vi "camera acquisition.vi"(0 "Interface Name":string="cam0", 9 "Stop (F)":bool, 11 "error in":errorcluster) -> (4 "Image Out":T1(plugin-control), 6 "Frame Rate":dbl, 8 "Image Number":u32, 10 "Stopped":bool, 15 "error out":errorcluster)   [LabVIEW 2020]
doc: "Creates, and edits acquisitions using the NI Vision Acquisition Express VI.\n\nThe NI Vision Acquisition Wizard is launched by placing the Express VI on the block diagram. Select an acquisition source and configure an acquisition using NI-IMAQ, NI-IMAQdx, or simulate an acquisition by reading an AVI or image files from a folder. After an acquisition is configured, select controls and indicators to be able to programmatically set in LabVIEW. Double-click the Vision Acquisition Express VI to edit the acquisition.\n\nNote: Any images created by the Express VI need to be disposed after use. Use the IMAQ Dispose.vi to cleanup the images output by the Express VI when they are no longer needed."
uses:
  <vilib>/vision/driver/NI_Vision_Acquisition_Software.lvlib
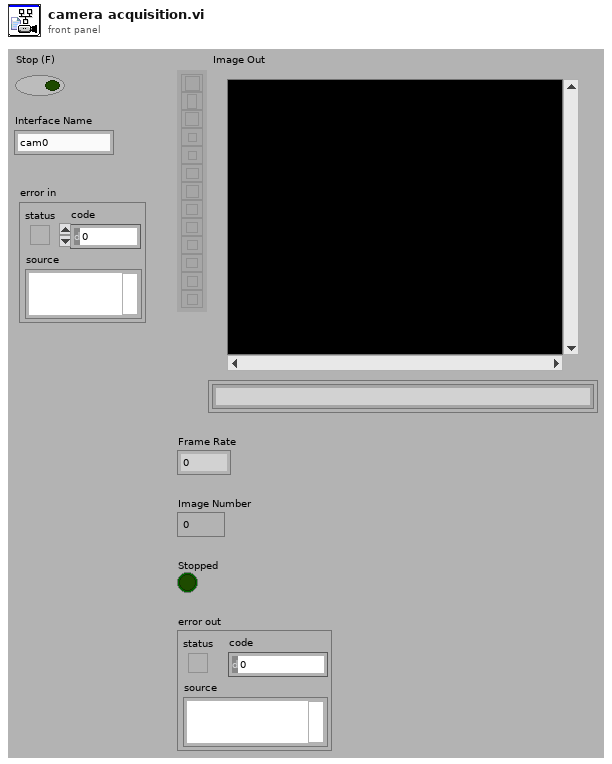
[diagram p1: front panel]
types:
  T1 = typedef "IMAQ Image.ctl" = refnum<image>
  T2 = typedef "IMAQdx.ctl" = refnum<k21>
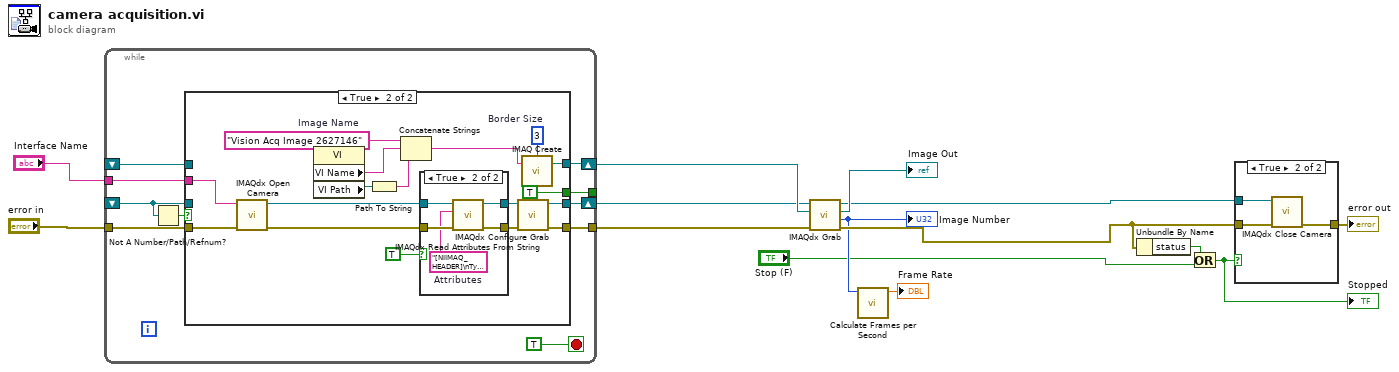
[diagram p0: block diagram]
diagram:
  n1 = while "While Loop_template0" {
    shift-right: [w24] -> w9
    shift-left: _ -> [w17]
    tunnel: [w23] -> w13
    tunnel: "error in" -> [w22]
    shift-right: [w20] -> w10
    shift-left: _ -> [w19]
    tunnel: "Interface Name" -> [w18]
    tunnel: [w15] -> _
    stop <- TRUE ("_template0") stop-if-true
    n2 = Not A Number/Path/Refnum?(number/path/refnum=w17) -> (NaN/Path/Refnum?=w16:bool)
    n3 = case "Case Structure_template0" shown="True" w16 {
      tunnel: [w27 w43] -> w24
      tunnel: w17 -> [w27 _]
      tunnel: [w26 w42] -> w23
      tunnel: w22 -> [w26 w44]
      tunnel: [w25 w41] -> w20
      tunnel: w19 -> [w25 _]
      tunnel: w18 -> [_ w31]
      tunnel: [_ TRUE] -> w15
      frame False {
      }
      frame True {
        w28 = 3  # Border Size
        w36 = "Vision Acq Image 2627146"  # Image Name
        n4 = call <vilib>:"IMAQdx Open Camera.vi"("error in"=w44, "Session In"=w31) -> ("error out"=w34:errorcluster, "Session Out"=w35:T2)  [unwired: 1 in, 7 out]
        n5 = property class="VI"() -> ("VI Name"=w39:string, "VI Path"=w40:path)  [unwired: 2 in, 2 out]
        n6 = Path To String(path=w40) -> (string=w38:string)
        n7 = Concatenate Strings(w36, w39, w38) -> (w37:string)
        n8 = case shown="True" TRUE ("Init Attributes") {
          tunnel: w35 -> [w46 w51]
          tunnel: w34 -> [w45 w50]
          tunnel: [w46 w48] -> w33
          tunnel: [w45 w47] -> w32
          frame False {
          }
          frame True {
            w49 = "[NIIMAQ_HEADER]\nType = 2\nVersion = 8\n\n[CAMERA_DATA]\nAcquisitionAttributes::Bayer::Algorithm = \"Bilinear\"\nAcquisitionAttributes::Bayer::GainB = \"1\"\nAcquisitionAttributes::Bayer::GainG = \"1\"\nAcquisitionAttributes::Bayer::GainR = \"1\"\nAcquisitionAttributes::Bayer::Pattern = \"Use hardware value\"\nAcquisitionAttributes::BitsPerPixel = \"Use hardware value\"\nAcquisitionAttributes::HardwareMaximumQueuedBufferCount = \"1000\"\nAcquisitionAttributes::HardwareRequeueBufferListThreshold = \"50\"\nAcquisitionAttributes::IgnoreFirstFrame = \"false\"\nAcquisitionAttributes::ImageDecoderCopyMode = \"Auto\"\nAcquisitionAttributes::OutputImageType = \"Auto\"\nAcquisitionAttributes::OverwriteMode = \"Get Newest\"\nAcquisitionAttributes::PixelSignedness = \"Use hardware value\"\nAcquisitionAttributes::ReceiveTimestampMode = \"None\"\nAcquisitionAttributes::ShiftPixelBits = \"false\"\nAcquisitionAttributes::SwapPixelBytes = \"false\"\nAcquisitionAttributes::Timeout = \"5000\"\nAcquisitionAttributes::VerticalMirror = \"false\"\nAcquisitionAttributes::VideoMode = \"640x480 YUY2 30.00fps\"\nCameraAttributes::BacklightCompensation::Mode = \"Manual\"\nCameraAttributes::BacklightCompensation::Value = \"true\"\nCameraAttributes::Brightness::Mode = \"Manual\"\nCameraAttributes::Brightness::Value = \"0\"\nCameraAttributes::Contrast::Mode = \"Manual\"\nCameraAttributes::Contrast::Value = \"0.179999999999999993\"\nCameraAttributes::Exposure::Mode = \"Auto\"\nCameraAttributes::Gain::Mode = \"Manual\"\nCameraAttributes::Gain::Value = \"1\"\nCameraAttributes::Gamma::Mode = \"Manual\"\nCameraAttributes::Gamma::Value = \"1.5\"\nCameraAttributes::Hue::Mode = \"Manual\"\nCameraAttributes::Hue::Value = \"0\"\nCameraAttributes::Saturation::Mode = \"Manual\"\nCameraAttributes::Saturation::Value = \"8\"\nCameraAttributes::Sharpness::Mode = \"Manual\"\nCameraAttributes::Sharpness::Value = \"3\"\nCameraAttributes::WhiteBalance::Mode = \"Auto\"\n"  # Attributes
            n9 = call <vilib>:"IMAQdx Read Attributes From String.vi"("error in"=w50, "Attributes String In"=w49, "Session In"=w51) -> ("error out"=w47:errorcluster, "Session Out"=w48:T2)  [unwired: 7 out]
          }
        }
        n10 = call <vilib>:"IMAQdx Configure Grab.vi"("error in"=w32, "Session In"=w33) -> ("error out"=w42:errorcluster, "Session Out"=w43:T2)  [unwired: 1 in, 7 out]
        n11 = call "IMAQ Create"("Border Size"=w28, "Image Name"=w37) -> ("New Image"=w41:T1)  [unwired: 2 in, 2 out]
      }
    }
  }
  n12 = call <vilib>:"IMAQdx Grab.vi"("error in"=w13, "Image In"=w10, "Session In"=w9) -> ("error out"=w8:errorcluster, "Buffer Number Out"=w7:u32, "Image Out"=→"Image Out":T1, "Session Out"=w5:T2)  [unwired: 1 in, 4 out]
  "Image Number" <- w7
  n13 = call <vilib>:"Calculate Frames per Second.vi"("Buffer Number"=w7) -> ("Acquired Frames/s"=→"Frame Rate":dbl)  [unwired: 2 in, 8 out]
  n14 = Unbundle By Name(w8) -> ("status"=w1:bool)
  n15 = Or(x=w1, y="Stop (F)") -> (x .or. y?=w2:bool)
  "Stopped" <- w2
  n16 = case "Case Structure_template1" shown="True" w2 {
    tunnel: [w52 w54] -> w4
    tunnel: w8 -> [w52 w55]
    tunnel: w5 -> [_ w53]
    frame False {
    }
    frame True {
      n17 = call <vilib>:"IMAQdx Close Camera.vi"("error in"=w55, "Session In"=w53) -> ("error out"=w54:errorcluster)  [unwired: 9 out]
    }
  }
  "error out" <- w4
